vi "Begin.vi"(8 "error in (no error)":errorcluster, 10 "Settings":variant, 11 "Pod Drive in":refnum<class "Pod Drive.lvclass">) -> (0 "error out":errorcluster, 3 "Pod Drive out":refnum<class "Pod Drive.lvclass">)   [LabVIEW 2019, in "DriveOld.lvlib" / "Pod Drive.lvclass"]
doc: "This VI holds the begin code"
uses:
  Pod Drive.lvclass
  <vilib>/Rock Robotics/WPI/SafetyOutput/WPI_SafetyOutputConfigMenu.ctl
  Pod Drive.lvclass/Pod Drive.ctl
  <vilib>/Rock Robotics/WPI/RobotDrive/WPI_RobotDriveOpen2MotorWithExistingMotors.vi
  Drive.lvclass
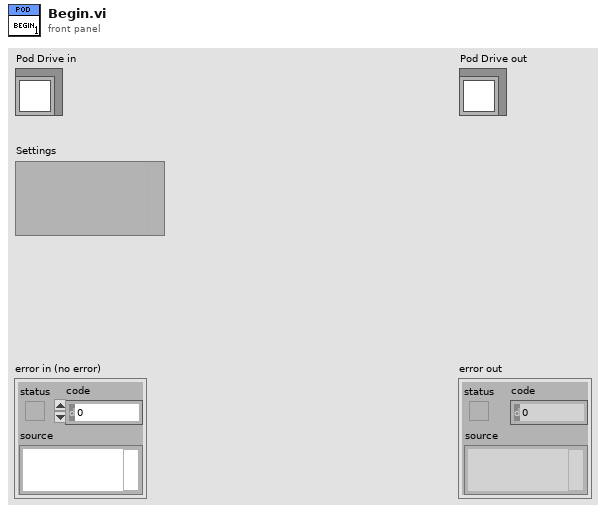
[diagram p1: front panel]
types:
  T1 = typedef "WPI_SafetyOutputConfigMenu.ctl" = enum16{"Enable", "Disable"}
  T2 = typedef "DriveOld.lvlib/Drive.lvclass/Drive Sensor Data.ctl" = cluster{"Drive Right Invert":bool, "Drive Right Sensor Phase":bool, "Drive Left Invert":bool, "Drive Left Sensor Phase":bool}
  T3 = typedef "WPI_MotorControlDeviceRef.ctl" = cluster{"DeviceStatus":errorcluster, "Type":T4, "PWM":cluster{"PWM Channel":T5, "DeadBand":T6}, "CAN":cluster{"Device Number":u8, "SetOutput VI Ref":variant, "GetOutput VI Ref":variant, "Enable VI Ref":variant, "Disable VI Ref":variant, "Data":variant}, "Invert":bool, "DIO PWM":cluster{"PWM \"Enable\" Channel":T5, "DIOChannel":T7, "PWM Rate":dbl}}
  T4 = typedef "WPI_MotorControlType.ctl" = enum16{"PWM", "CAN", "DIO PWM"}
  T5 = typedef "FPGA_DIOPWMChannel.ctl" = enum8{"PWM 0", "PWM 1", "PWM 2", "PWM 3", "PWM 4", "PWM 5", "PWM 6", "PWM 7", "PWM 8", "PWM 9", "PWM MXP 0", "PWM MXP 1", "PWM MXP 2", "PWM MXP 3", "PWM MXP 4", "PWM MXP 5", "PWM MXP 6", "PWM MXP 7", "PWM MXP 8", "PWM MXP 9", "Invalid"}
  T6 = typedef "WPI_PWMDeadband.ctl" = cluster{"Name":string, "maxPositivePwm":i32, "minPositivePwm":i32, "centerPwm":i32, "maxNegativePwm":i32, "minNegativePwm":i32, "angularRange":u16}
  T7 = typedef "FPGA_DIOChannel.ctl" = enum8{"DIO 0", "DIO 1", "DIO 2", "DIO 3", "DIO 4", "DIO 5", "DIO 6", "DIO 7", "DIO 8", "DIO 9", "DIO MXP 0", "DIO MXP 1", "DIO MXP 2", "DIO MXP 3", "DIO MXP 4", "DIO MXP 5", "DIO MXP 6", "DIO MXP 7", "DIO MXP 8", "DIO MXP 9", "DIO MXP 10", "DIO MXP 11", "DIO MXP 12", "DIO MXP 13", "DIO MXP 14", "DIO MXP 15", "SPI Port CS1", "SPI Port CS2", "SPI Port CS3", "SPI Port MISO", "SPI Port MOSI", "Invalid"}
  T8 = typedef "WPI_RobotDriveDevRef.ctl" = cluster{"DevStatus":errorcluster, "Motors[]":T3[], "Square Inputs":bool, "Max Output":dbl}
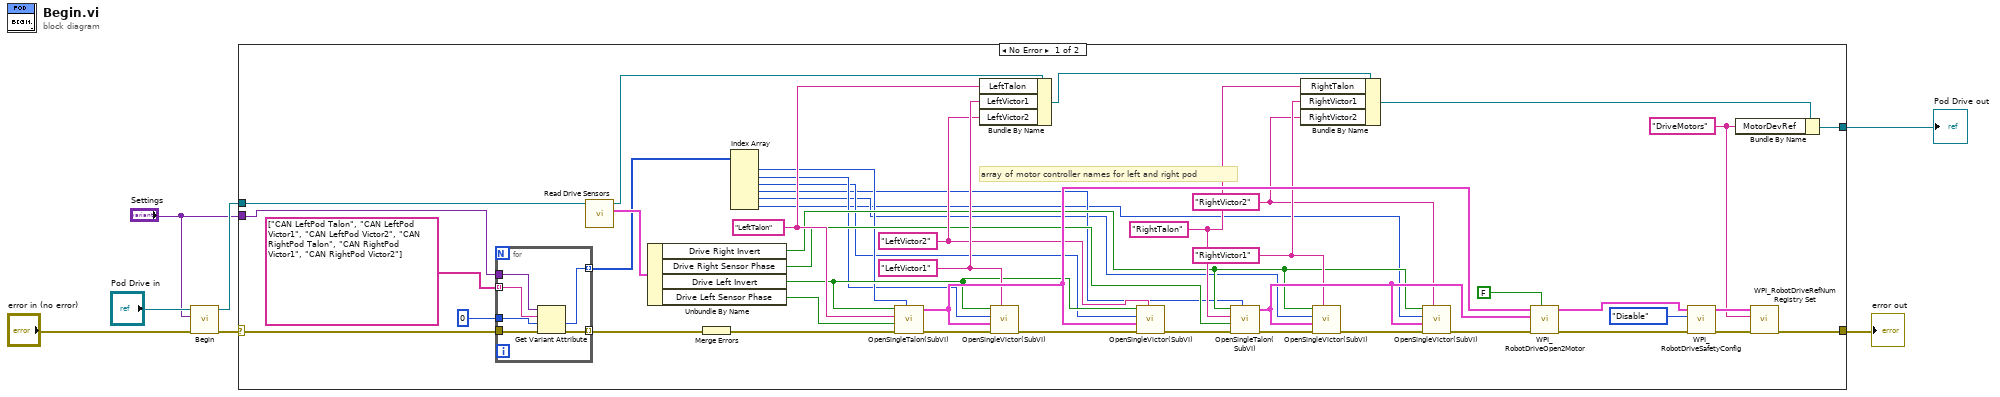
[diagram p0: block diagram]
diagram:
  n1 = call-parent "Begin.vi"("error in (no error)"="error in (no error)", "Settings"="Settings", "Drive in"="Pod Drive in") -> ("error out"=w5:errorcluster, "Drive out"=w4:refnum<class "Pod Drive.lvclass">)  [unwired: 7 in]
  n2 = case shown="No Error" w5 {
    selector: w5 -> [w20 w60]
    tunnel: [w28 w60] -> w7
    tunnel: [w31 w59] -> w2
    tunnel: w4 -> [w8 w59]
    tunnel: "Settings" -> [w21 _]
    frame No Error {
      w33 = "RightVictor2" ("RightVictor2")
      w34 = "RightVictor1" ("RightVictor1")
      w40 = "DriveMotors" ("refnum name")
      w30 = "RightTalon" ("RightTalon")
      w42 = "LeftVictor2" ("LeftVictor2")
      w43 = "LeftVictor1" ("LeftVictor1")
      w29 = "LeftTalon" ("LeftTalon")
      # "array of motor controller names for left and right pod"
      n3 = for {
        tunnel: w21 -> [w58]
        tunnel: w20 -> [w57]
        tunnel: [w56] -> w19 mode=indexing
        tunnel: u8 0 ("Talon") -> [w55]
        tunnel: string[] ["CAN LeftPod Talon", "CAN LeftPod Victor1", "CAN LeftPod Victor2", "CAN RightPod Talon", "CAN RightPod Victor1", "CAN RightPod Victor2"] -> [w54] mode=indexing
        tunnel: [w53] -> w15 mode=indexing
        n4 = Get Variant Attribute(Variant=w58, name=w54, default value (empty Variant)=w55, error in=w57) -> (value=w53:u8, error out=w56:errorcluster)  [unwired: 2 out]
      }
      n5 = call-dynamic "Read Drive Sensors.vi"("Drive in"=w8) -> ("Drive Sensors"=w26:T2, "Drive out"=w27:refnum<class "Pod Drive.lvclass">)  [unwired: 8 in, 1 out]
      n6 = Unbundle By Name(w26) -> ("Drive Right Invert"=w22:bool, "Drive Right Sensor Phase"=w24:bool, "Drive Left Invert"=w23:bool, "Drive Left Sensor Phase"=w25:bool)
      n7 = Merge Errors(w19) -> (w18:errorcluster)
      n8 = Index Array(array=w15) -> (element #1=w14:u8, element #2=w13:u8, element #3=w12:u8, element #4=w11:u8, element #5=w10:u8, element #6=w9:u8)  [unwired: 6 in]
      n9 = call "OpenSingleTalon(SubVI).vi"("can_id"=w14, "error in (no error)"=w18, "sensor_phase"=w25, "refnum name"=w29, "invert"=w23) -> ("error out"=w46:errorcluster, "PhoenixMotorControlDevRef"=w44:T3)  [unwired: 5 in]
      n10 = Bundle By Name(cluster=w27, "LeftTalon"=w29, "LeftVictor1"=w43, "LeftVictor2"=w42) -> (w41:refnum<class "Pod Drive.lvclass">)
      n11 = call "OpenSingleVictor(SubVI).vi"("refnum name"=w43, "error in (no error)"=w46, "Master Controller to Follow"=w44, "Device Number"=w13, "Invert?"=w23) -> ("error out"=w45:errorcluster)  [unwired: 5 in, 1 out]
      n12 = call "OpenSingleVictor(SubVI).vi"("refnum name"=w42, "error in (no error)"=w45, "Master Controller to Follow"=w44, "Device Number"=w12, "Invert?"=w23) -> ("error out"=w38:errorcluster)  [unwired: 5 in, 1 out]
      n13 = call "OpenSingleTalon(SubVI).vi"("can_id"=w11, "error in (no error)"=w38, "sensor_phase"=w24, "refnum name"=w30, "invert"=w22) -> ("error out"=w37:errorcluster, "PhoenixMotorControlDevRef"=w35:T3)  [unwired: 5 in]
      n14 = Bundle By Name(cluster=w41, "RightTalon"=w30, "RightVictor1"=w34, "RightVictor2"=w33) -> (w39:refnum<class "Pod Drive.lvclass">)
      n15 = call "OpenSingleVictor(SubVI).vi"("refnum name"=w34, "error in (no error)"=w37, "Master Controller to Follow"=w35, "Device Number"=w10, "Invert?"=w22) -> ("error out"=w36:errorcluster)  [unwired: 5 in, 1 out]
      n16 = call "OpenSingleVictor(SubVI).vi"("refnum name"=w33, "error in (no error)"=w36, "Master Controller to Follow"=w35, "Device Number"=w9, "Invert?"=w22) -> ("error out"=w32:errorcluster)  [unwired: 5 in, 1 out]
      n17 = call-poly <vilib>:"WPI_RobotDriveOpen2Motor.vi"("Square Inputs"=FALSE, "error in (no error)"=w32, "Right Motor Dev Ref"=w35, "Left Motor Dev Ref"=w44) -> ("error out"=w52:errorcluster, "RobotDriveDevRef"=w50:T8)  [unwired: 6 in]
      n18 = call <vilib>:"WPI_RobotDriveSafetyConfig.vi"("error in (no error)"=w52, "mode"=WPI_SafetyOutputConfigMenu."Disable", "RobotDriveDevRef"=w50) -> ("error out"=w51:errorcluster, "RobotDriveDevRef"=w49:T8)  [unwired: 7 in]
      n19 = Bundle By Name(cluster=w39, "MotorDevRef"=w40) -> (w31:refnum<class "Pod Drive.lvclass">)
      n20 = call <vilib>:"WPI_RobotDriveRefNum Registry Set.vi"("error in (no error)"=w51, "refnum name"=w40, "RobotDriveDevRef"=w49) -> ("error out"=w28:errorcluster)  [unwired: 7 in, 1 out]
    }
    frame Error {
    }
  }
  "error out" <- w7
  "Pod Drive out" <- w2
